vi "Write MultiBand.vi"(8 "error in (no error)":errorcluster, 10 "MultiBand":T2(array[cluster]), 11 "MultiBandState in":refnum<class "MultiBandState.lvclass">) -> (0 "error out":errorcluster, 3 "MultiBandState out":refnum<class "MultiBandState.lvclass">)   [LabVIEW 2018, in "Functions.lvlib" / "MultiBandState.lvclass"]
uses:
  MultiBandState.lvclass
  <vilib>/Analysis/Matrix/Datatypes/RealMatrix.ctl
  MultiBandState.lvclass/MultiBandState.ctl
  <vilib>/Analysis/Matrix/NI_Matrix.lvlib
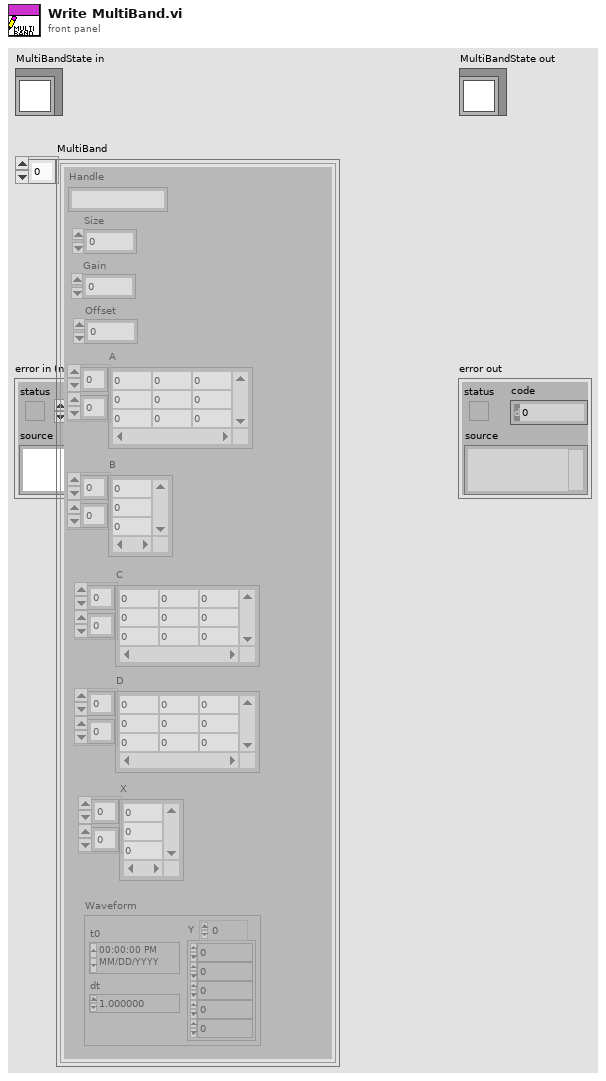
[diagram p1: front panel]
types:
  T1 = typedef "NI_Matrix.lvlib/RealMatrix.ctl" = dbl[][]
  T2 = cluster{"Handle":string, "Size":i32, "Gain":dbl, "Offset":dbl, "A":T1, "B":T1, "C":T1, "D":T1, "X":T1, "Waveform":waveform(dbl)}[]
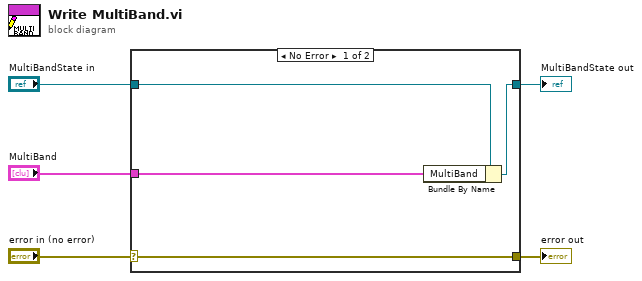
[diagram p0: block diagram]
diagram:
  n1 = case shown="No Error" "error in (no error)" {
    selector: "error in (no error)" -> [w9 w10]
    tunnel: [w9 w10] -> w4
    tunnel: [w7 w11] -> w2
    tunnel: "MultiBandState in" -> [w8 w11]
    tunnel: "MultiBand" -> [w6 _]
    frame No Error {
      n2 = Bundle By Name(cluster=w8, "MultiBand"=w6) -> (w7:refnum<class "MultiBandState.lvclass">)
    }
    frame Error {
    }
  }
  "error out" <- w4
  "MultiBandState out" <- w2
